vi "Begin.vi"(8 "error in (no error)":errorcluster, 10 "Config In":variant, 11 "Tank Drive in":refnum<class "Tank Drive.lvclass">) -> (0 "error out":errorcluster, 3 "Tank Drive out":refnum<class "Tank Drive.lvclass">)   [LabVIEW 2019, in "Drive.lvlib" / "Tank Drive.lvclass"]
uses:
  Tank Drive.lvclass
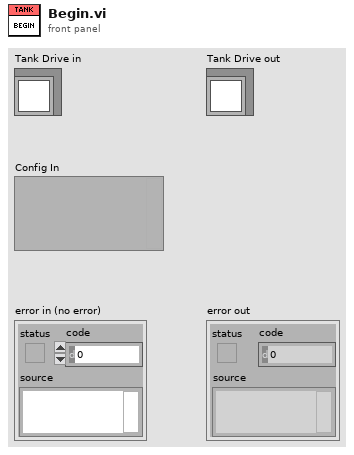
[diagram p1: front panel]
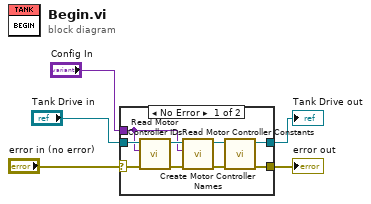
[diagram p0: block diagram]
diagram:
  n1 = case shown="No Error" "error in (no error)" {
    selector: "error in (no error)" -> [w14 w16]
    tunnel: [w8 w16] -> w4
    tunnel: [w6 w15] -> w2
    tunnel: "Tank Drive in" -> [w13 w15]
    tunnel: "Config In" -> [w9 _]
    frame No Error {
      n2 = call "Read Motor Controller IDs.vi"("error in (no error)"=w14, "settings in"=w9, "Tank Drive in"=w13) -> ("error out"=w10:errorcluster, "Tank Drive out"=w11:refnum<class "Tank Drive.lvclass">)  [unwired: 7 in]
      n3 = call "Read Motor Controller Constants.vi"("error in (no error)"=w10, "settings in"=w9, "Tank Drive in"=w11) -> ("error out"=w12:errorcluster, "Tank Drive out"=w7:refnum<class "Tank Drive.lvclass">)  [unwired: 7 in]
      n4 = call "Create Motor Controller Names.vi"("error in (no error)"=w12, "Tank Drive in"=w7) -> ("error out"=w8:errorcluster, "Tank Drive out"=w6:refnum<class "Tank Drive.lvclass">)  [unwired: 8 in]
    }
    frame Error {
    }
  }
  "error out" <- w4
  "Tank Drive out" <- w2
